vi "LifeTimeImagePoint.vi"(0 "Boolean in":refnum<vi>, 1 "Bool Refnum":refnum<vi>, 2 "reference 5":refnum<vi>, 3 "String":string, 4 "reference 6":refnum<vi>, 5 "String 2":string, 6 "reference 7":refnum<vi>, 7 "error in (no error)":errorcluster, 8 "reference 4":refnum<vi>, 9 "reference 8":refnum<vi>, 10 "reference 3":refnum<vi>, 11 "reference 9":refnum<vi>, 12 "reference in":refnum<vi>, 13 "DigNum Refnum":refnum<vi>, 14 "Numeric in":i32, 15 "Str Refnum":refnum<vi>, 16 "X Stepsize":dbl, 18 "Array in":i32[][](array[numeric]), 19 "Point Measurement":refnum<vi>) -> (20 "Array out":i32[][](array[numeric]), 21 "CCD Chip Size":i32, 22 "X Start":dbl, 23 "Numeric out":dbl, 27 "error out":errorcluster)   [LabVIEW 2013]
uses:
  Camera/lib/Examples/LabVIEW/System Files/user.lib/atmcd32d.llb/Error Code Enum typedef.ctl
  Camera/vi/ccdChipPixels.vi
  Camera/vi/CamDef.vi
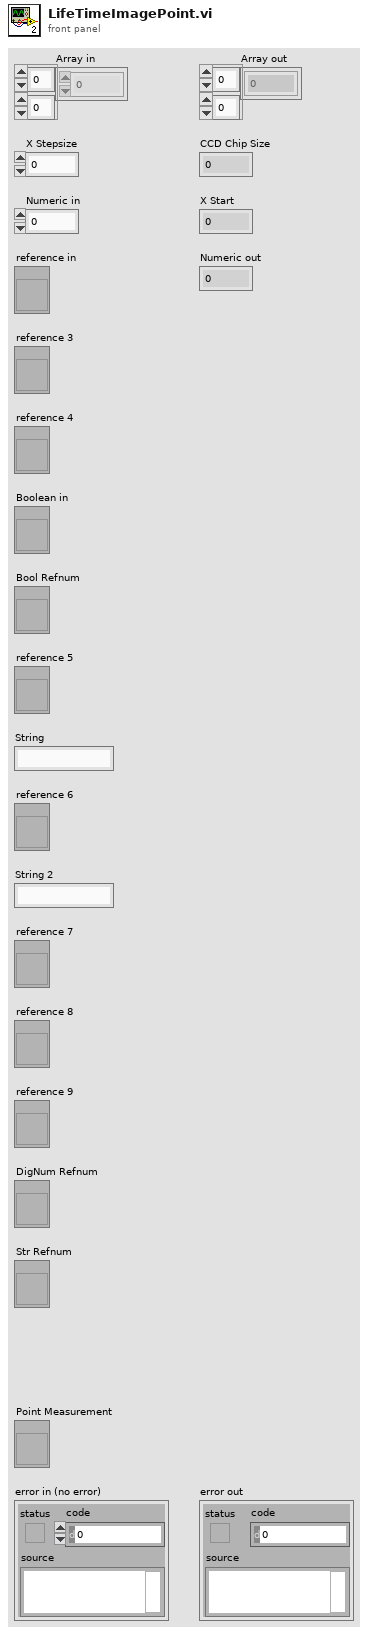
[diagram p1: front panel]
types:
  T1 = enum16{"No Measurement", "Aquire Image", "Point Measurement", "Multi Measurement", "Save Color Image"}
  T2 = enum16{"No Measurement", "Aquire Image", "Point Measurement", "Multi Measurement", "Save Color Image", "Find Single Mol.", "Auto Measurement Control", "Auto Point", "Aquire Line Scan", "Grid Measurement", "Trapping", "Move Scanner"}
  T3 = typedef "Error Code Enum typedef.ctl" = enum32{"N/A (0)", "DRV_ERROR_CODES", "DRV_SUCCESS", "DRV_VXDNOTINSTALLED", "DRV_ERROR_SCAN", "DRV_ERROR_CHECK_SUM", "DRV_ERROR_FILELOAD", "DRV_UNKNOWN_FUNC", "DRV_ERROR_VXD_INIT", "DRV_ERROR_ADDRESS", "DRV_ERROR_PAGELOCK", "DRV_ERROR_PAGEUNLOCK", "DRV_ERROR_BOARDTEST", "DRV_ERROR_ACK", "DRV_ERROR_UP_FIFO", "DRV_ERROR_PATTERN", "N/A (16)", "DRV_ACQUISITION_ERRORS", "DRV_ACQ_BUFFER", "DRV_ACQ_DOWNFIFO_FULL", "DRV_PROC_UNKONWN_INSTRUCTION", "DRV_ILLEGAL_OP_CODE", "DRV_KINETIC_TIME_NOT_MET", "DRV_ACCUM_TIME_NOT_MET", "DRV_NO_NEW_DATA", "N/A (25)", "DRV_SPOOLERROR", "N/A (27)", "N/A (28)", "N/A (29)", "N/A (30)", "N/A (31)", "N/A (32)", "DRV_TEMPERATURE_CODES", "DRV_TEMPERATURE_OFF", "DRV_TEMPERATURE_NOT_STABILIZED", "DRV_TEMPERATURE_STABILIZED", "DRV_TEMPERATURE_NOT_REACHED", "DRV_TEMPERATURE_OUT_RANGE", "DRV_TEMPERATURE_NOT_SUPPORTED", "DRV_TEMPERATURE_DRIFT", "N/A (41)", "N/A (42)", "N/A (43)", "N/A (44)", "N/A (45)", "N/A (46)", "N/A (47)", "N/A (48)", "DRV_GENERAL_ERRORS", "DRV_INVALID_AUX", "DRV_COF_NOTLOADED", "DRV_FPGAPROG", "DRV_FLEXERROR", "DRV_GPIBERROR", "N/A (55)", "N/A (56)", "N/A (57)", "N/A (58)", "N/A (59)", "N/A (60)", "N/A (61)", "N/A (62)", "N/A (63)", "DRV_DATATYPE", "DRV_DRIVER_ERRORS", "DRV_P1INVALID", "DRV_P2INVALID", "DRV_P3INVALID", "DRV_P4INVALID", "DRV_INIERROR", "DRV_COFERROR", "DRV_ACQUIRING", "DRV_IDLE", "DRV_TEMPCYCLE", "DRV_NOT_INITIALIZED", "DRV_P5INVALID", "DRV_P6INVALID", "DRV_INVALID_MODE", "DRV_INVALID_FILTER", "DRV_I2CERRORS", "DRV_I2CDEVNOTFOUND", "DRV_I2CTIMEOUT", "DRV_P7INVALID", "N/A (84)", "N/A (85)", "N/A (86)", "N/A (87)", "N/A (88)", "N/A (89)", "DRV_IOCERROR", "DRV_VRMVERSIONERROR"}
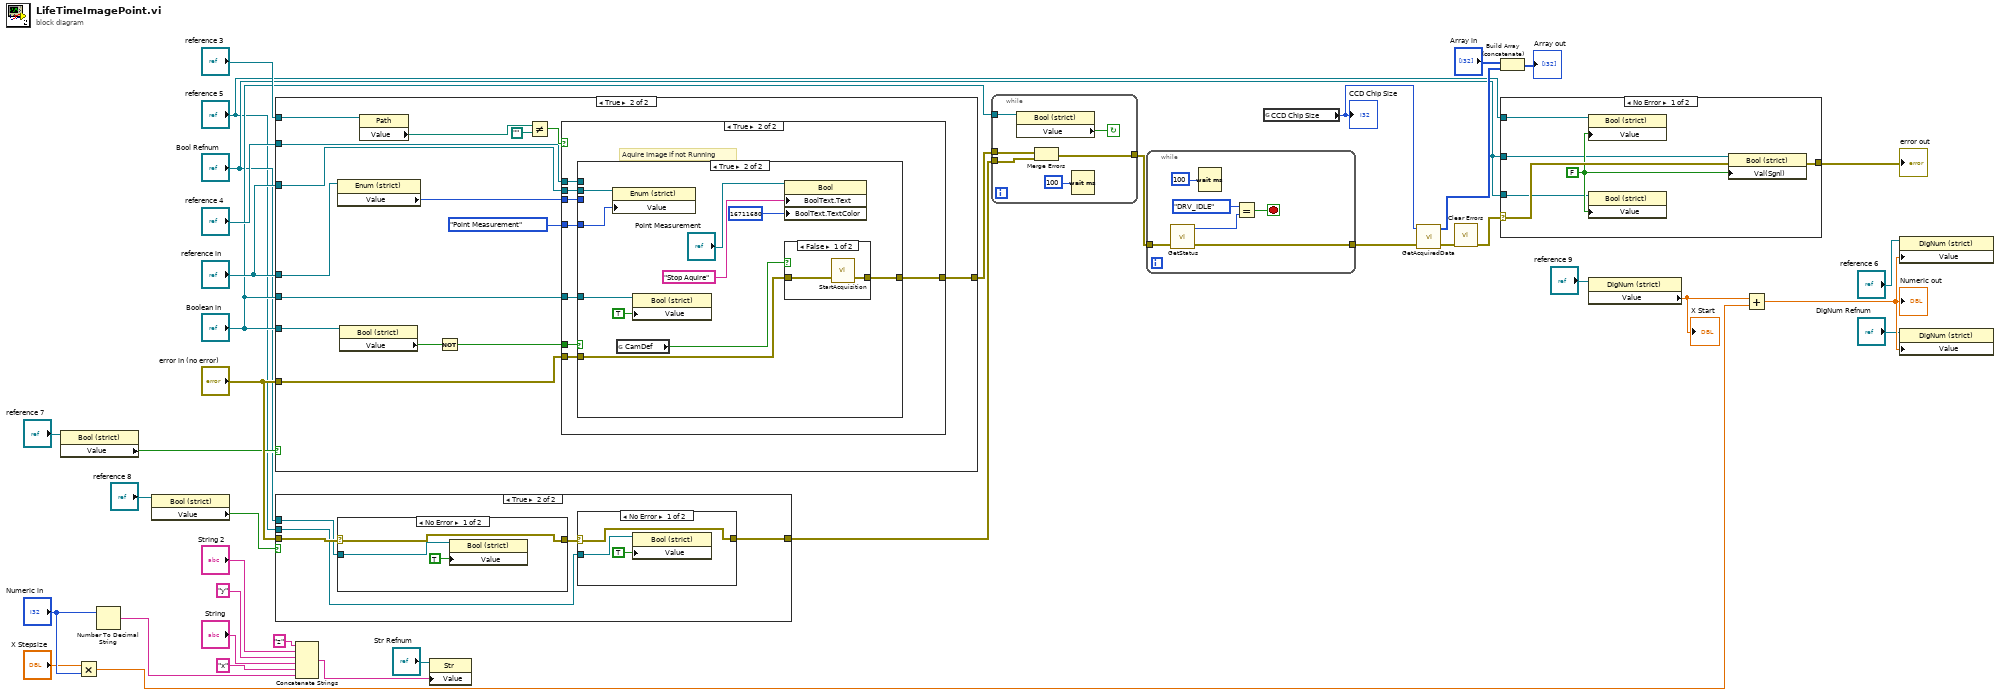
[diagram p0: block diagram]
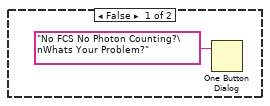
[diagram p6: hidden frame]
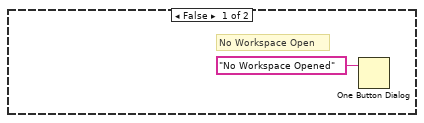
[diagram p7: hidden frame]
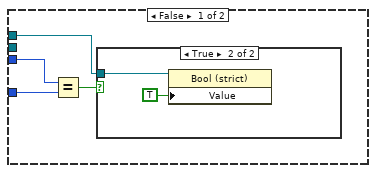
[diagram p8: hidden frame]
diagram:
  n1 = property class="Bool (strict)"(reference="reference 7") -> ("Value"=w24:bool)  [unwired: 1 in, 2 out]
  n2 = Multiply(x="X Stepsize", y="Numeric in") -> (x*y=w26:dbl)
  n3 = Number To Decimal String(number="Numeric in") -> (decimal integer string=w21:string)  [unwired: 1 in]
  n4 = property class="Bool (strict)"(reference="reference 8") -> ("Value"=w25:bool)  [unwired: 1 in, 2 out]
  n5 = case shown="True" w24 {
    tunnel: [_ w48] -> w13
    tunnel: "error in (no error)" -> [_ w47]
    tunnel: "Boolean in" -> [_ w45]
    tunnel: "reference in" -> [_ w44]
    tunnel: "reference 3" -> [_ w43]
    tunnel: "reference 4" -> [_ w42]
    tunnel: "reference in" -> [_ w41]
    tunnel: "Boolean in" -> [_ w40]
    frame False {
      n6 = One Button Dialog(message="No FCS No Photon Counting?\nWhats Your Problem?") -> ()  [unwired: 1 in, 1 out]
    }
    frame True {
      n7 = property class="Enum (strict)"(reference=w44) -> ("Value"=w53:T2)  [unwired: 1 in, 2 out]
      n8 = property class="Bool (strict)"(reference=w45) -> ("Value"=w54:bool)  [unwired: 1 in, 2 out]
      n9 = property class="Path"(reference=w43) -> ("Value"=w46:path)  [unwired: 1 in, 2 out]
      n10 = Not(x=w54) -> (.not. x?=w49:bool)
      n11 = Not Equal?(x=w46, y=path "") -> (x != y?=w50:bool)
      n12 = case shown="True" w50 {
        tunnel: w49 -> [_ w63]
        tunnel: T1."Point Measurement" ("Do Measurement") -> [_ w62]
        tunnel: w53 -> [_ w61]
        tunnel: [_ w60] -> w48
        tunnel: w47 -> [_ w59]
        tunnel: w42 -> [_ w58]
        tunnel: w41 -> [_ w57]
        tunnel: w40 -> [_ w56]
        frame False {
          # "No Workspace Open"
          n13 = One Button Dialog(message="No Workspace Opened") -> ()  [unwired: 1 in, 1 out]
        }
        frame True {
          # "Aquire Image if not Running"
          n14 = case shown="True" w63 {
            tunnel: w62 -> [w66 w77]
            tunnel: w61 -> [w67 _]
            tunnel: [_ w74] -> w60
            tunnel: w59 -> [_ w73]
            tunnel: w58 -> [w64 _]
            tunnel: w57 -> [_ w71]
            tunnel: w56 -> [_ w70]
            frame False {
              n15 = Equal?(x=w67, y=w66) -> (x = y?=w65:bool)
              n16 = case shown="True" w65 {
                tunnel: w64 -> [_ w68]
                frame False {
                }
                frame True {
                  n17 = property class="Bool (strict)"(reference=w68, "Value"=TRUE ("Stop Measurement")) -> ()  [unwired: 1 in, 2 out]
                }
              }
            }
            frame True {
              n18 = property class="Enum (strict)"(reference=w71, "Value"=w77) -> ()  [unwired: 1 in, 2 out]
              n19 = global read "CamDef.vi" "CamDef"() -> (w72:bool)
              n20 = property class="Bool (strict)"(reference=w70, "Value"=TRUE ("Measurement Running")) -> ()  [unwired: 1 in, 2 out]
              n21 = property on="Property Node" class="Bool"(reference="Point Measurement", "BoolText.Text"="Stop Aquire" ("Caption.Text"), "BoolText.TextColor"=u32 16711680 ("Boolean Text.Colors:FG Color")) -> ()  [unwired: 1 in, 2 out]
              n22 = case shown="False" w72 {
                tunnel: [w80 w82] -> w74
                tunnel: w73 -> [w81 w82]
                frame False {
                  n23 = call "StartAcquisition.vi"("error in (no error)"=w81) -> ("error out"=w80:errorcluster)  [unwired: 1 in, 1 out]
                }
                frame True {
                }
              }
            }
          }
        }
      }
    }
  }
  n24 = case shown="True" w25 {
    tunnel: [w83 w87] -> w23
    tunnel: "error in (no error)" -> [w83 w86]
    tunnel: "Bool Refnum" -> [_ w85]
    tunnel: "reference 5" -> [_ w84]
    frame False {
    }
    frame True {
      n25 = case shown="No Error" w86 {
        selector: w86 -> [w94 _]
        tunnel: [w94 _] -> w88
        tunnel: w85 -> [w92 _]
        frame No Error {
          n26 = property class="Bool (strict)"(reference=w92, "Value"=TRUE ("Trap")) -> ()  [unwired: 1 in, 2 out]
        }
        frame Error {
        }
      }
      n27 = case shown="No Error" w88 {
        selector: w88 -> [w91 _]
        tunnel: [w91 _] -> w87
        tunnel: w84 -> [w89 _]
        frame No Error {
          n28 = property class="Bool (strict)"(reference=w89, "Value"=TRUE ("Record")) -> ()  [unwired: 1 in, 2 out]
        }
        frame Error {
        }
      }
    }
  }
  n29 = Concatenate Strings("z" ("string"), "String 2", "y" ("string"), "String", "x" ("string"), w21) -> (w38:string)
  n30 = property on="Property Node" class="Str"(reference="Str Refnum", "Value"=w38) -> ()  [unwired: 1 in, 2 out]
  n31 = while {
    tunnel: w13 -> [w98]
    tunnel: w23 -> [w97]
    tunnel: [w96] -> w29
    tunnel: "Boolean in" -> [w95]
    stop <- w100 continue-if-true
    n32 = property class="Bool (strict)"(reference=w95) -> ("Value"=w100:bool)  [unwired: 1 in, 2 out]
    n33 = Merge Errors(w98, w97) -> (w96:errorcluster)
    n34 = Wait (ms)(milliseconds to wait=u32 100) -> ()  [unwired: 1 out]
  }
  n35 = while {
    tunnel: w29 -> [w101]
    tunnel: [w104] -> w28
    stop <- w103 stop-if-true
    n36 = call "GetStatus.vi"("error in (no error)"=w101) -> ("error out"=w104:errorcluster, "status"=w105:T3)  [unwired: 2 in, 1 out]
    n37 = Wait (ms)(milliseconds to wait=u32 100) -> ()  [unwired: 1 out]
    n38 = Equal?(x=Error_Code_Enum_typedef."DRV_IDLE" ("status"), y=w105) -> (x = y?=w103:bool)
  }
  n39 = global read "ccdChipPixels.vi" "CCD Chip Size"() -> (w36:i32)
  "CCD Chip Size" <- w36
  n40 = call "GetAcquiredData.vi"("error in (no error)"=w28, "size"=w36) -> ("error out"=w30:errorcluster, "array"=w32:i32[])  [unwired: 1 in, 1 out]
  n41 = call <vilib>:"Clear Errors.vi"("error in (no error)"=w30) -> ("error out"=w31:errorcluster)  [unwired: 6 in]
  n42 = Build Array (concatenate)("Array in", w32) -> (→"Array out":i32[][])
  n43 = case shown="No Error" w31 {
    selector: w31 -> [w111 w113]
    tunnel: [w112 w113] -> w22
    tunnel: "Bool Refnum" -> [w109 _]
    tunnel: "reference 5" -> [w108 _]
    tunnel: "Bool Refnum" -> [w107 _]
    frame No Error {
      w110 = FALSE ("Value (Signaling)")
      n44 = property class="Bool (strict)"(reference=w108, "Value"=w110) -> ()  [unwired: 1 in, 2 out]
      n45 = property class="Bool (strict)"(reference=w107, "Value"=w110) -> ()  [unwired: 1 in, 2 out]
      n46 = property on="Property Node" class="Bool (strict)"(reference=w109, error in=w111, "Val(Sgnl)"=w110) -> (error out=w112:errorcluster)  [unwired: 1 out]
    }
    frame Error {
    }
  }
  "error out" <- w22
  n47 = property class="DigNum (strict)"(reference="reference 9") -> ("Value"=w35:dbl)  [unwired: 1 in, 2 out]
  "X Start" <- w35
  n48 = Add(x=w35, y=w26) -> (x+y=w37:dbl)
  "Numeric out" <- w37
  n49 = property class="DigNum (strict)"(reference="reference 6", "Value"=w37) -> ()  [unwired: 1 in, 2 out]
  n50 = property on="Property Node" class="DigNum (strict)"(reference="DigNum Refnum", "Value"=w37) -> ()  [unwired: 1 in, 2 out]
